vi "Add ClientID Session.vi"(8 "error in (no error)":errorcluster, 9 "SessionMailbox":refnum<queue>, 10 "Client ID":string, 11 "Server in":refnum<class "Server.lvclass">) -> (0 "error out":errorcluster, 3 "Server out":refnum<class "Server.lvclass">)   [LabVIEW 2013, in "MQTT Server.lvlib" / "Server.lvclass"]
uses:
  Server.lvclass
  MQTT_Base/Response -- cluster.ctl
  Control Packets/ControlPacket/ControlPacket.lvclass
  Server.lvclass/Server.ctl
  MQTT_Base/MQTT_Base.lvclass
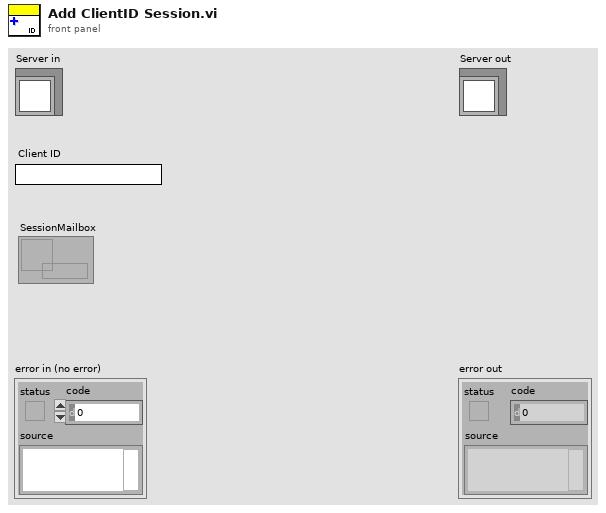
[diagram p1: front panel]
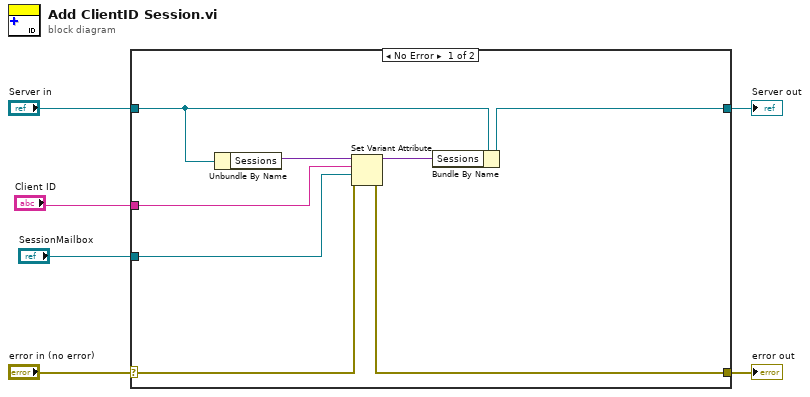
[diagram p0: block diagram]
diagram:
  n1 = case shown="No Error" "error in (no error)" {
    selector: "error in (no error)" -> [w11 w16]
    tunnel: [w10 w16] -> w5
    tunnel: [w7 w15] -> w3
    tunnel: "Server in" -> [w8 w15]
    tunnel: "Client ID" -> [w13 _]
    tunnel: "SessionMailbox" -> [w12 _]
    frame No Error {
      n2 = Unbundle By Name(w8) -> ("Sessions"=w14:variant)
      n3 = Set Variant Attribute(Variant=w14, name=w13, value=w12, error in=w11) -> (Variant out=w9:variant, error out=w10:errorcluster)  [unwired: 1 out]
      n4 = Bundle By Name(cluster=w8, "Sessions"=w9) -> (w7:refnum<class "Server.lvclass">)
    }
    frame Error {
    }
  }
  "error out" <- w5
  "Server out" <- w3
